vi "mupLibPath.vi"() -> (2 "libmuparser path":path=path "muparser-2.2.5/lib/libmuparser.so.2.2.4:")   [LabVIEW 2018, in "mupLib.lvlib"]
doc: "Build path constant of the muParser shared library based on OS and bitness."
uses:
  mupLib.lvlib
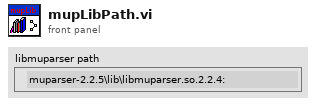
[diagram p1: front panel]
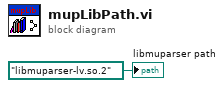
[diagram p0: block diagram]
diagram:
  "libmuparser path" <- path "libmuparser-lv.so.2" ("libmuparser path")
